vi "FGV Gasdefinition.vi"(6 "Aktion":T1, 8 "error in (no error)":errorcluster caption="Fehler (Eingang, kein Fehler)", 11 "Gas":string) -> (0 "error out":errorcluster caption="Fehler (Ausgang)", 3 "Gase":string[](array[string]))   [LabVIEW 2020, in "System Einstellungen V2.lvlib"]
uses:
  System Einstellungen V2.lvlib
  Aktion FGV Gasdefinition.ctl
  Allgemein/allgemeine Sub-VIs.lvlib
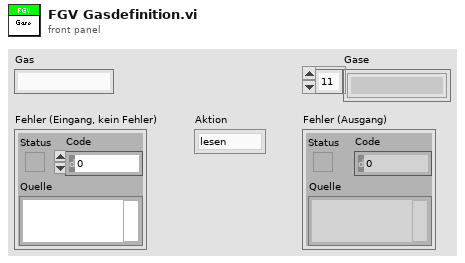
[diagram p1: front panel]
types:
  T1 = typedef "System Einstellungen V2.lvlib/Aktion FGV Gasdefinition.ctl" = enum16{"lesen", "schreiben", "löschen", "laden", "speichern"}
  T2 = enum16{"open", "replace", "create", "open or create", "replace or create", "replace or create with confirmation"}
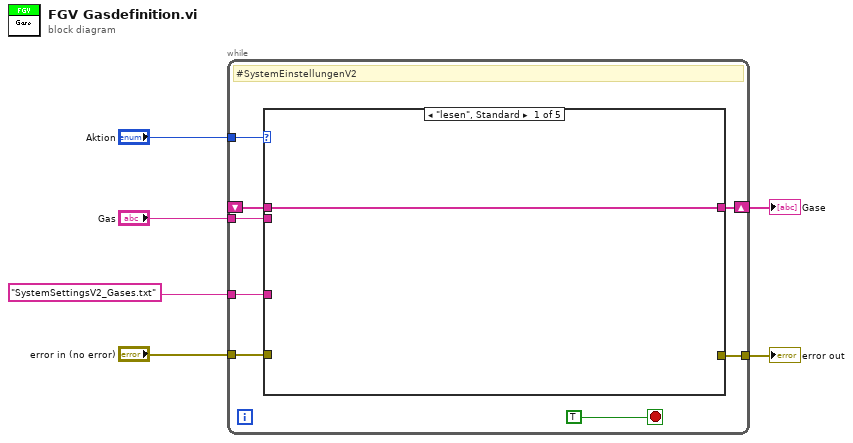
[diagram p0: block diagram]
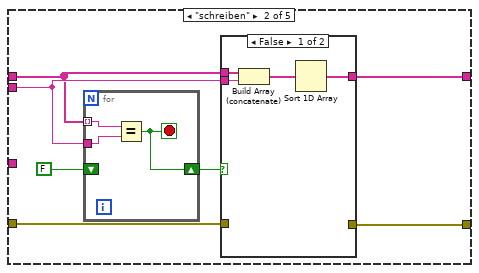
[diagram p2: hidden frame]
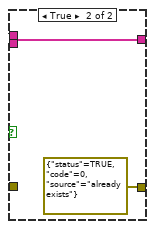
[diagram p3: hidden frame]
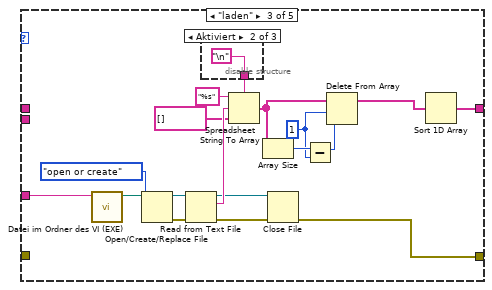
[diagram p4: hidden frame]
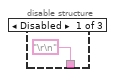
[diagram p5: hidden frame]
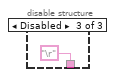
[diagram p6: hidden frame]
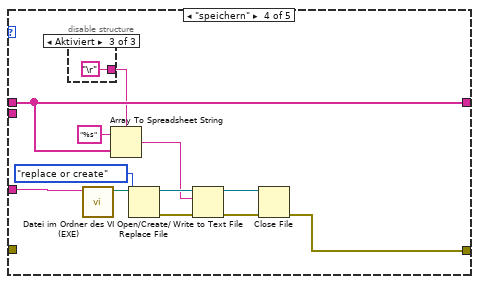
[diagram p7: hidden frame]
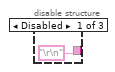
[diagram p8: hidden frame]
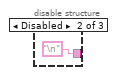
[diagram p9: hidden frame]
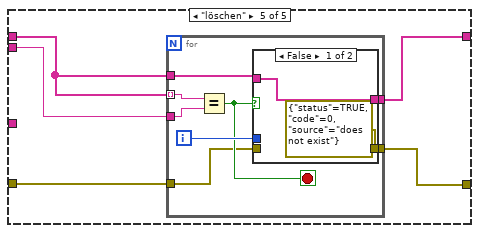
[diagram p10: hidden frame]
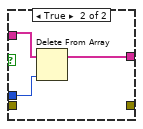
[diagram p11: hidden frame]
diagram:
  n1 = while {
    tunnel: "Aktion" -> [w13]
    shift-right: [w12] -> w5
    shift-left: _ -> [w11]
    tunnel: "Gas" -> [w10]
    tunnel: "SystemSettingsV2_Gases.txt" ("Dateiname") -> [w9]
    tunnel: "error in (no error)" -> [w8]
    tunnel: [w7] -> w1
    stop <- TRUE stop-if-true
    # "#SystemEinstellungenV2"
    n2 = case shown="\"lesen\", Standard" w13 {
      tunnel: [w15 w22 w33 w55 w70] -> w12
      tunnel: w11 -> [w15 w20 _ w55 w71]
      tunnel: w10 -> [_ w21 _ _ w72]
      tunnel: w9 -> [_ _ w49 w63 _]
      tunnel: w8 -> [_ w17 _ _ w69]
      tunnel: [_ w16 w32 w53 w68] -> w7
      frame "lesen", Default {
      }
      frame "schreiben" {
        n3 = for {
          tunnel: w20 -> [w31] mode=indexing
          tunnel: w21 -> [w30]
          shift-right: [w29] -> w18
          shift-left: FALSE -> [_]
          stop <- w29 stop-if-true
          n4 = Equal?(x=w31, y=w30) -> (x = y?=w29:bool)
        }
        n5 = case shown="False" w18 {
          tunnel: [w23 w28] -> w22
          tunnel: w20 -> [w26 w28]
          tunnel: w21 -> [w25 _]
          tunnel: w17 -> [_ _]
          tunnel: [_ errorcluster {"status"=TRUE, "code"=0, "source"="already exists"} ("error in (no error)")] -> w16
          frame False {
            n6 = Build Array (concatenate)(w26, w25) -> (w24:string[])
            n7 = Sort 1D Array(array=w24) -> (sorted array=w23:string[])
          }
          frame True {
          }
        }
      }
      frame "laden" {
        w35 = 1 ("x")
        n8 = call "Datei im Ordner des VI (EXE).vi"("Dateiname"=w49) -> ("Dateipfad im Ordner des Haupt-VIs"=w48:path)  [unwired: 8 in, 2 out]
        n9 = Open/Create/Replace File(file path (use dialog)=w48, operation (0:open)=T2."open or create" ("Operation (0:open)")) -> (refnum out=w46:refnum<file>, error out=w47:errorcluster)  [unwired: 4 in, 1 out]
        n10 = Read from Text File(file (use dialog)=w46, error in=w47) -> (refnum out=w43:refnum<file>, text=w45:string, error out=w42:errorcluster)  [unwired: 2 in, 1 out]
        n11 = disable-structure shown="Aktiviert" {
          disable-tunnel: ["\r\n" "\n" "\r"] -> w39
          frame Disabled {
          }
          frame Enabled {
          }
          frame Disabled {
          }
        }
        n12 = Spreadsheet String To Array(delimiter (Tab)=w39, format string="%s" ("Format-String"), spreadsheet string=w45, array type (2D Dbl)=string[] []) -> (array=w37:string[])
        n13 = Array Size(array=w37) -> (size(s)=w38:i32)
        n14 = Close File(refnum=w43, error in=w42) -> (error out=w32:errorcluster)  [unwired: 1 out]
        n15 = Subtract(x=w38, y=w35) -> (x-y=w36:i32)
        n16 = Delete From Array(array=w37, length=w35, index=w36) -> (array with subset deleted=w34:string[])  [unwired: 1 out]
        n17 = Sort 1D Array(array=w34) -> (sorted array=w33:string[])
      }
      frame "speichern" {
        n18 = disable-structure shown="Aktiviert" {
          disable-tunnel: ["\r\n" "\n" "\r"] -> w54
          frame Disabled {
          }
          frame Disabled {
          }
          frame Enabled {
          }
        }
        n19 = call "Datei im Ordner des VI (EXE).vi"("Dateiname"=w63) -> ("Dateipfad im Ordner des Haupt-VIs"=w64:path)  [unwired: 8 in, 2 out]
        n20 = Array To Spreadsheet String(delimiter (Tab)=w54, array=w55, 3:"%s" ("Format-String")) -> (spreadsheet string=w58:string)
        n21 = Open/Create/Replace File(file path (use dialog)=w64, operation (0:open)=T2."replace or create" ("Operation (0:open)")) -> (refnum out=w62:refnum<file>, error out=w61:errorcluster)  [unwired: 4 in, 1 out]
        n22 = Write to Text File(file (use dialog)=w62, text=w58, error in=w61) -> (refnum out=w59:refnum<file>, error out=w60:errorcluster)  [unwired: 1 in, 1 out]
        n23 = Close File(refnum=w59, error in=w60) -> (error out=w53:errorcluster)  [unwired: 1 out]
      }
      frame "löschen" {
        n24 = for {
          tunnel: w71 -> [w80] mode=indexing
          tunnel: w72 -> [w79]
          tunnel: w71 -> [w78]
          tunnel: [w76] -> w70
          tunnel: w69 -> [w74]
          tunnel: [w73] -> w68
          i -> [w77]
          stop <- w75 stop-if-true
          n25 = Equal?(x=w80, y=w79) -> (x = y?=w75:bool)
          n26 = case shown="False" w75 {
            tunnel: w78 -> [w82 w85]
            tunnel: w77 -> [_ w84]
            tunnel: [w82 w83] -> w76
            tunnel: w74 -> [_ _]
            tunnel: [errorcluster {"status"=TRUE, "code"=0, "source"="does not exist"} ("error in (no error)") _] -> w73
            frame False {
            }
            frame True {
              n27 = Delete From Array(array=w85, index=w84) -> (array with subset deleted=w83:string[])  [unwired: 1 in, 1 out]
            }
          }
        }
      }
    }
  }
  "Gase" <- w5
  "error out" <- w1
